vi "tempRegulator.vi"() -> ()   [LabVIEW 2021]
panel:
  out "?":dbl
  in  "Atmospheric Temperature":dbl(slide) scale=0.0..100.0
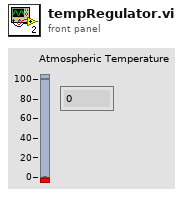
[diagram p1: front panel]
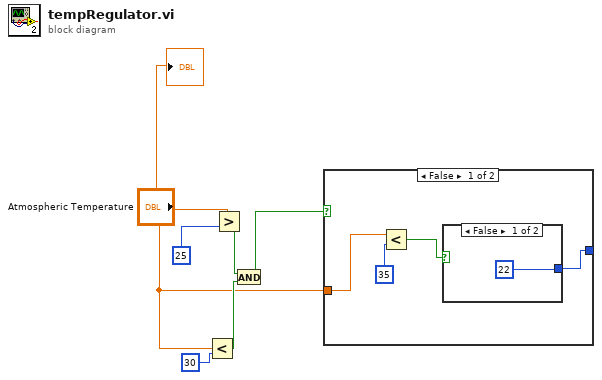
[diagram p0: block diagram]
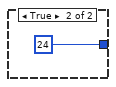
[diagram p2: hidden frame]
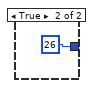
[diagram p3: hidden frame]
diagram:
  n1 = Less?(x="Atmospheric Temperature", y=30) -> (x < y?=w3:bool)
  n2 = Greater?(x="Atmospheric Temperature", y=25) -> (0:w4:bool)
  n3 = And(x=w4, y=w3) -> (x .and. y?=w2:bool)
  n4 = case shown="False" w2 {
    tunnel: [w7 26] -> _
    tunnel: "Atmospheric Temperature" -> [w10 _]
    frame False {
      n5 = Less?(x=w10, y=35) -> (x < y?=w8:bool)
      n6 = case shown="False" w8 {
        tunnel: [22 24] -> w7
        frame False {
        }
        frame True {
        }
      }
    }
    frame True {
    }
  }
  "?" <- "Atmospheric Temperature"
